vi "commande.vi"() -> ()   [LabVIEW 2015]
uses:
  <vilib>/httpClient/LabVIEWHTTPClient.lvlib
panel:
  in  "OK Button 8":bool
  in  "OK Button 3":bool
  in  "OK Button 2":bool
  in  "OK Button":bool
  in  "Combo Box 2":string(combo)
  in  "Combo Box":string(combo)
  # "Choisir  chambre"
  # "Choisir équipement"
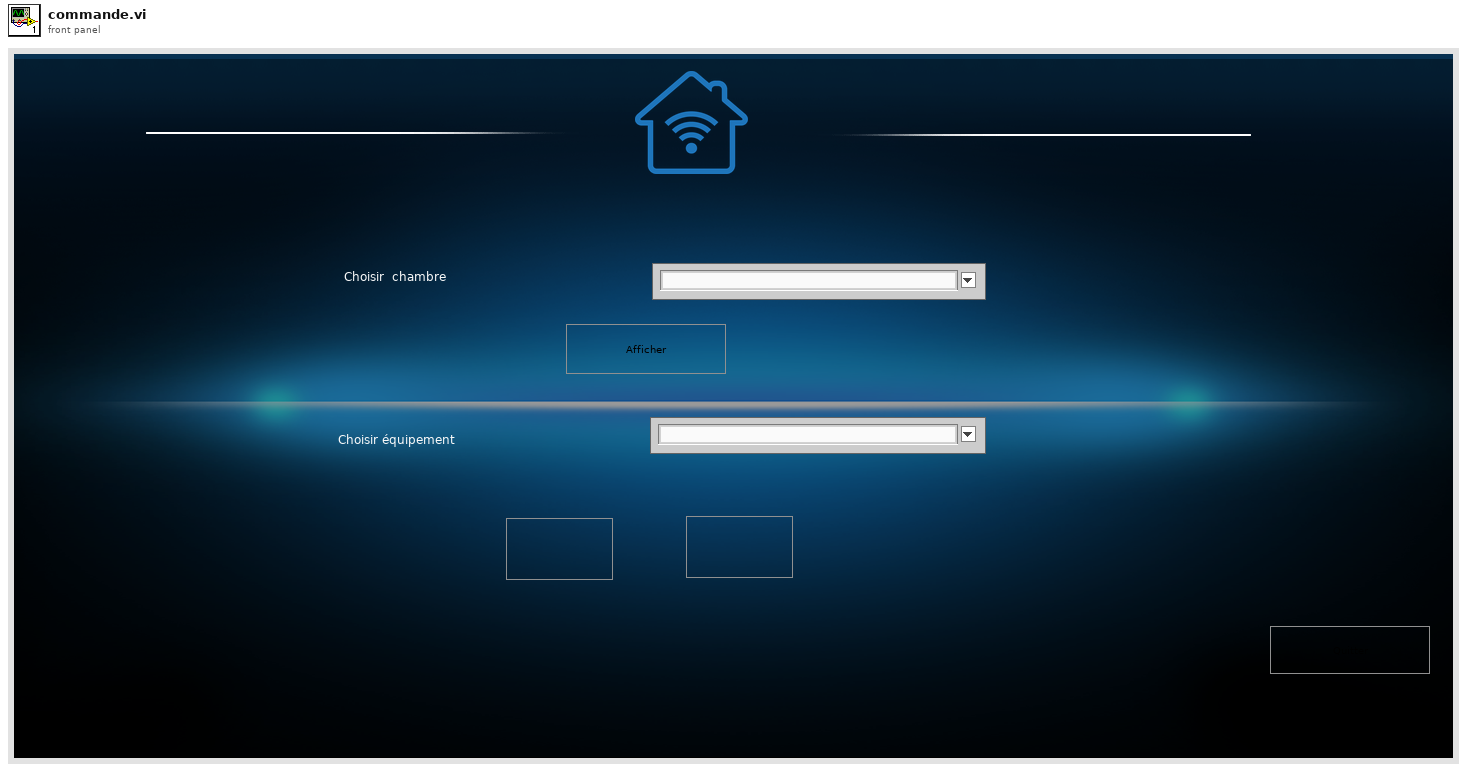
[diagram p1: front panel]
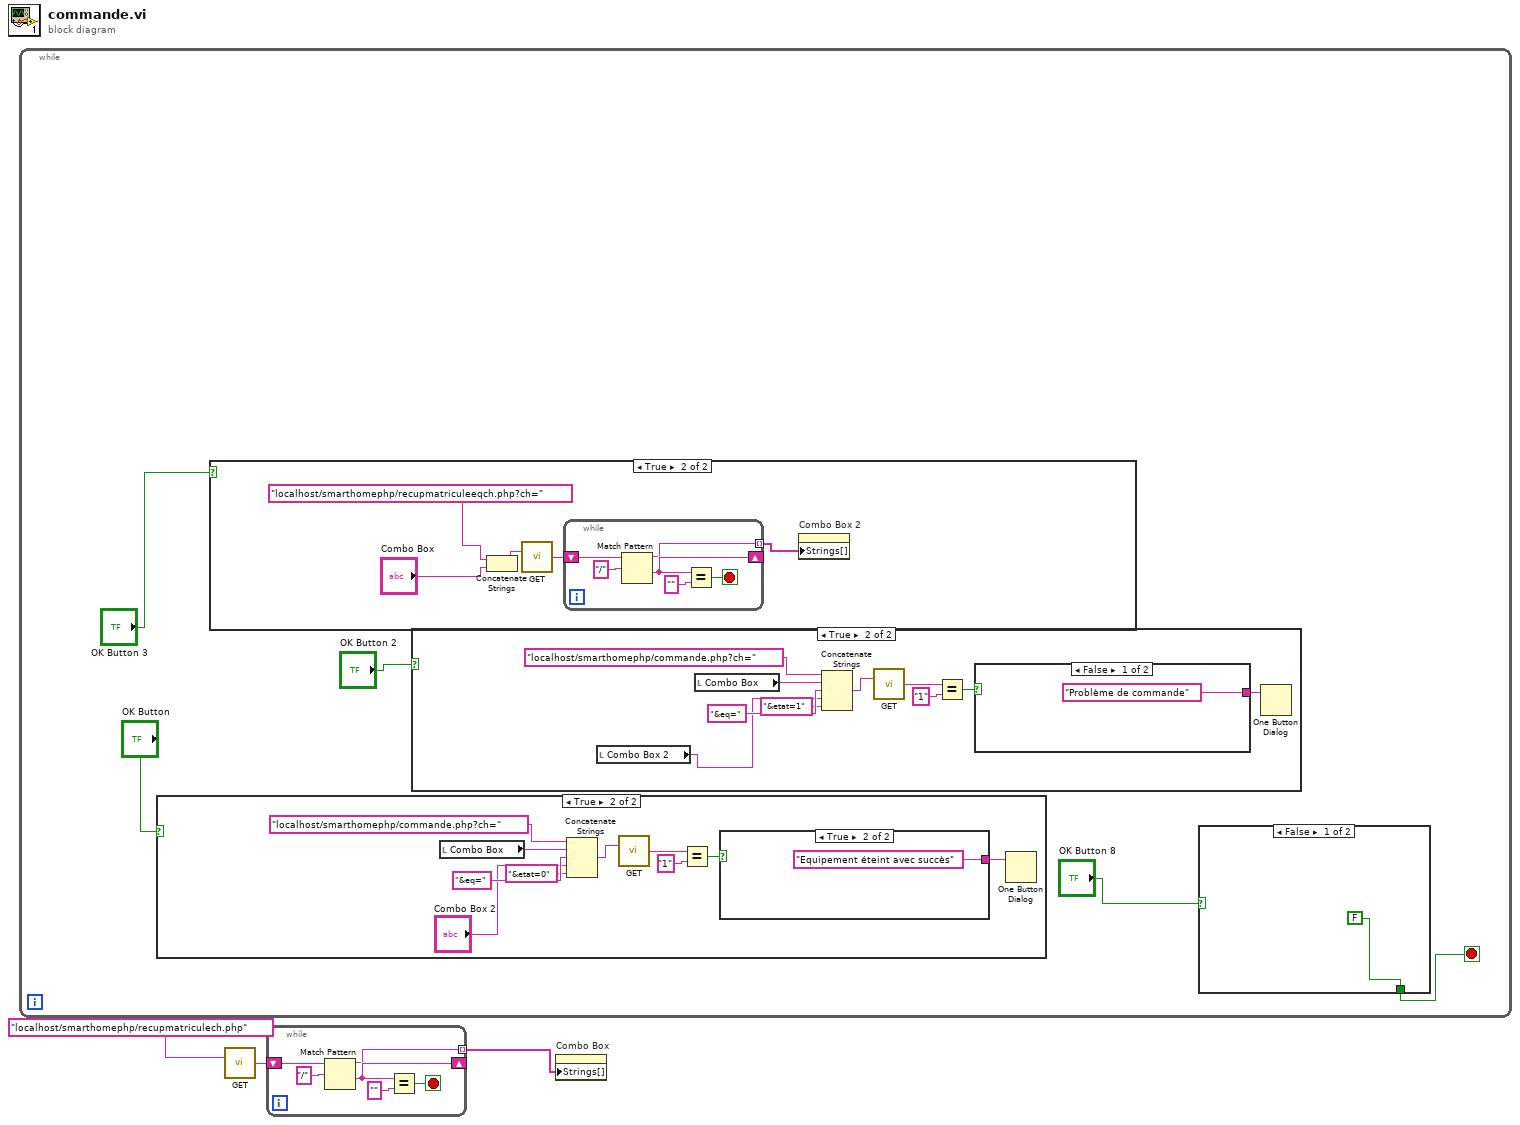
[diagram p0: block diagram]
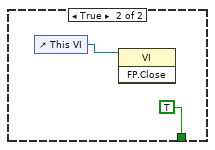
[diagram p2: hidden frame]
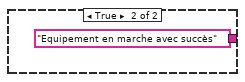
[diagram p4: hidden frame]
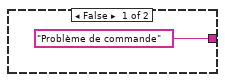
[diagram p6: hidden frame]
diagram:
  n1 = while {
    stop <- w4 stop-if-true
    n2 = case shown="True" "OK Button" {
      frame False {
      }
      frame True {
        n3 = local read "Combo Box"() -> (w28:string)
        n4 = Concatenate Strings("localhost/smarthomephp/commande.php?ch=", w28, "&eq=", "Combo Box 2", "&etat=0" ("string")) -> (w27:string)
        n5 = call <vilib>:"GET.vi"("url"=w27) -> ("body"=w30:string)  [unwired: 11 in, 3 out]
        n6 = Equal?(x=w30, y="1") -> (x = y?=w32:bool)
        n7 = case shown="True" w32 {
          tunnel: ["Problème de commande" "Equipement éteint avec succès"] -> w33
          frame False {
          }
          frame True {
          }
        }
        n8 = One Button Dialog(message=w33) -> ()  [unwired: 1 in, 1 out]
      }
    }
    n9 = case shown="True" "OK Button 3" {
      frame False {
      }
      frame True {
        n10 = Concatenate Strings("localhost/smarthomephp/recupmatriculeeqch.php?ch=", "Combo Box") -> (w36:string)
        n11 = call <vilib>:"GET.vi"("url"=w36) -> ("body"=w40:string)  [unwired: 11 in, 3 out]
        n12 = while {
          shift-right: [w43] -> _
          shift-left: w40 -> [w45]
          tunnel: [w41] -> w39 mode=indexing
          stop <- w42 stop-if-true
          n13 = Match Pattern(string=w45, regular expression="/") -> (before substring=w41:string, after substring=w43:string)  [unwired: 1 in, 2 out]
          n14 = Equal?(x=w43, y="") -> (x = y?=w42:bool)
        }
        n15 = property on="Combo Box 2" class="CmbBox"("Strings[]"=w39) -> ()  [unwired: 2 in, 2 out]
      }
    }
    n16 = case shown="True" "OK Button 2" {
      frame False {
      }
      frame True {
        n17 = local read "Combo Box 2"() -> (w12:string)
        n18 = local read "Combo Box"() -> (w16:string)
        n19 = Concatenate Strings("localhost/smarthomephp/commande.php?ch=", w16, "&eq=", w12, "&etat=1" ("string")) -> (w15:string)
        n20 = call <vilib>:"GET.vi"("url"=w15) -> ("body"=w18:string)  [unwired: 11 in, 3 out]
        n21 = Equal?(x=w18, y="1") -> (x = y?=w20:bool)
        n22 = case shown="False" w20 {
          tunnel: ["Problème de commande" "Equipement en marche avec succès"] -> w21
          frame False {
          }
          frame True {
          }
        }
        n23 = One Button Dialog(message=w21) -> ()  [unwired: 1 in, 1 out]
      }
    }
    n24 = case shown="False" "OK Button 8" {
      tunnel: [FALSE TRUE] -> w4
      frame False {
      }
      frame True {
        n25 = control-ref of="This VI"() -> (w11:refnum<vi>)
        n26 = invoke class="VI" method="FP.Close"(reference=w11) -> ()  [unwired: 2 in, 3 out]
      }
    }
  }
  n27 = call <vilib>:"GET.vi"("url"="localhost/smarthomephp/recupmatriculech.php") -> ("body"=w2:string)  [unwired: 11 in, 3 out]
  n28 = while {
    shift-right: [w49] -> _
    shift-left: w2 -> [w51]
    tunnel: [w47] -> w1 mode=indexing
    stop <- w48 stop-if-true
    n29 = Match Pattern(string=w51, regular expression="/") -> (before substring=w47:string, after substring=w49:string)  [unwired: 1 in, 2 out]
    n30 = Equal?(x=w49, y="") -> (x = y?=w48:bool)
  }
  n31 = property on="Combo Box" class="CmbBox"("Strings[]"=w1) -> ()  [unwired: 2 in, 2 out]
